vi "Parse Xml Node Recursively from File.vi"(6 "VI Data":T1[](array[typedef]), 8 "error in":errorcluster, 9 "Parents":string[](array[string]), 10 "Path to XML document":path caption="Path to Item LV XML Document") -> (0 "error out":errorcluster, 2 "VI Data out":T1[](array[typedef]))   [LabVIEW 2020, in "VI Properties Editor.lvlib"]
doc: "This VI is meant to be used to parse xml files like classes and lvlib that are nested members of a lvlib or one of it's members."
uses:
  VI Properties Editor.lvlib
  <vilib>/xml/NI_XML.lvlib
  <vilib>/xml/Load XML String.vi
  <vilib>/xml/Close Reference(Node).vi
  <vilib>/picture/picture.llb/imagedata.ctl
  CTLs/VI Properties.ctl
  CTLs/Control Properties.ctl
  CTLs/VI Data.ctl
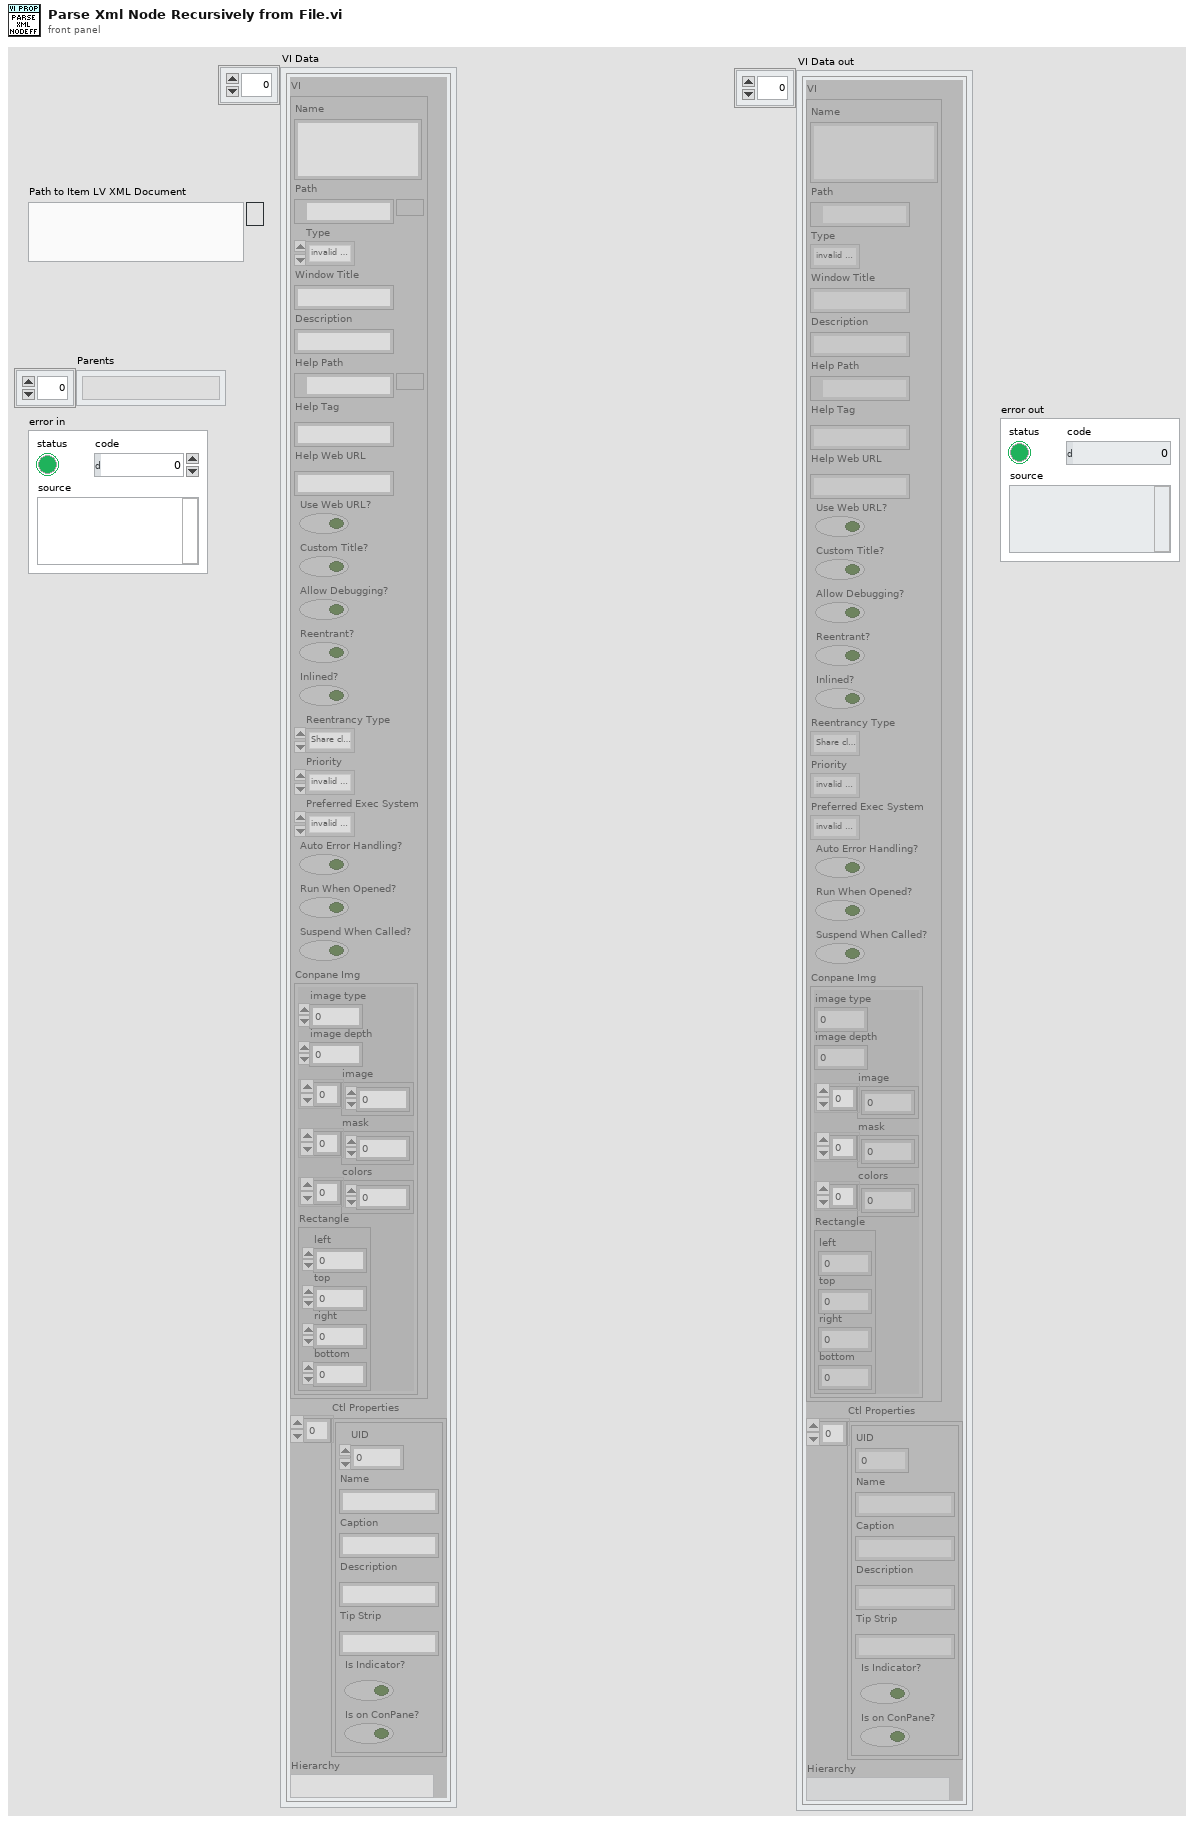
[diagram p1: front panel]
types:
  T1 = typedef "VI Properties Editor.lvlib/VI Data.ctl" = cluster{"VI":T2, "Ctl Properties":T4[], "Hierarchy":string}
  T2 = typedef "VI Properties Editor.lvlib/VI Properties.ctl" = cluster{"Name":string, "Path":path, "Type":enum32{"invalid VI type", "Standard VI", "Control VI", "Global VI", "Polymorphic VI", "Configuration VI", "SubSystem", "Facade VI", "Method VI", "Statechart Diagram VI"}, "Window Title":string, "Description":string, "Help Path":path, "Help Tag":string, "Help Web URL":string, "Use Web URL?":bool, "Custom Title?":bool, "Allow Debugging?":bool, "Reentrant?":bool, "Inlined?":bool, "Reentrancy Type":enum16{"Share clones between instances", "Preallocate clone for each instance"}, "Priority":enum32{"invalid priority", "background priority", "normal priority", "above normal priority", "high priority", "time critical priority", "subroutine"}, "Preferred Exec System":enum32{"invalid execution system", "user interface", "standard", "instrument i/o", "data acquisition", "other 1", "other 2", "same as caller"}, "Auto Error Handling?":bool, "Run When Opened?":bool, "Suspend When Called?":bool, "Conpane Img":T3}
  T3 = typedef "imagedata.ctl" = cluster{"image type":i32, "image depth":i32, "image":u8[], "mask":u8[], "colors":u32[], "Rectangle":cluster{"left":i16, "top":i16, "right":i16, "bottom":i16}}
  T4 = typedef "VI Properties Editor.lvlib/Control Properties.ctl" = cluster{"UID":i32, "Name":string, "Caption":string, "Description":string, "Tip Strip":string, "Is Indicator?":bool, "Is on ConPane?":bool}
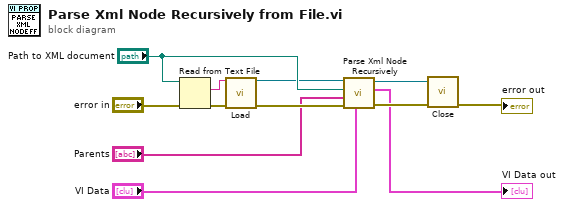
[diagram p0: block diagram]
diagram:
  n1 = Read from Text File(file (use dialog)="Path to XML document", error in="error in") -> (text=w10:string, error out=w11:errorcluster)  [unwired: 2 in, 2 out]
  n2 = call-poly <vilib>:"Load.vi"("XML string"=w10, "error in (no error)"=w11) -> ("DOM document out"=w7:refnum<k20>, "error out"=w8:errorcluster)  [unwired: 11 in, 1 out]
  n3 = call "Parse Xml Node Recursively.vi"("VI Data"="VI Data", "error in"=w8, "Parents"="Parents", "XML File Path"="Path to XML document", "Node in"=w7) -> ("error out"=w6:errorcluster, "VI Data out"=→"VI Data out":T1[], "Node out"=w1:refnum<k20>)  [unwired: 4 in]
  n4 = call-poly <vilib>:"Close.vi"("error in (no error)"=w6, "node"=w1) -> ("error out"=→"error out":errorcluster)  [unwired: 7 in]
